vi "get_stage_position.vi"(8 "error IN":errorcluster, 11 "reference IN":refnum<k7>) -> (0 "error OUT":errorcluster, 2 "Stage position OUT":T1, 3 "reference OUT":refnum<k7>)   [LabVIEW 2020]
uses:
  typedefs/typedef_stage_position.ctl
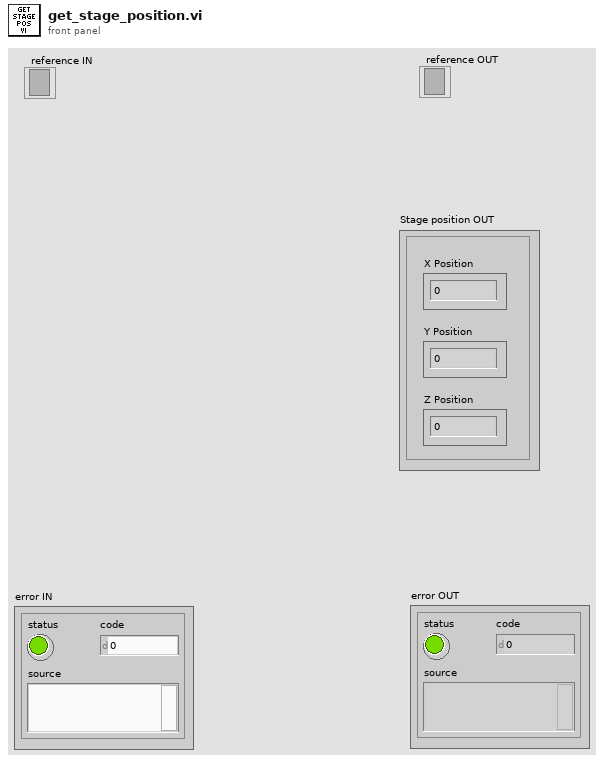
[diagram p1: front panel]
types:
  T1 = typedef "typedef_stage_position.ctl" = cluster{"X Position":dbl, "Y Position":dbl, "Z Position":dbl}
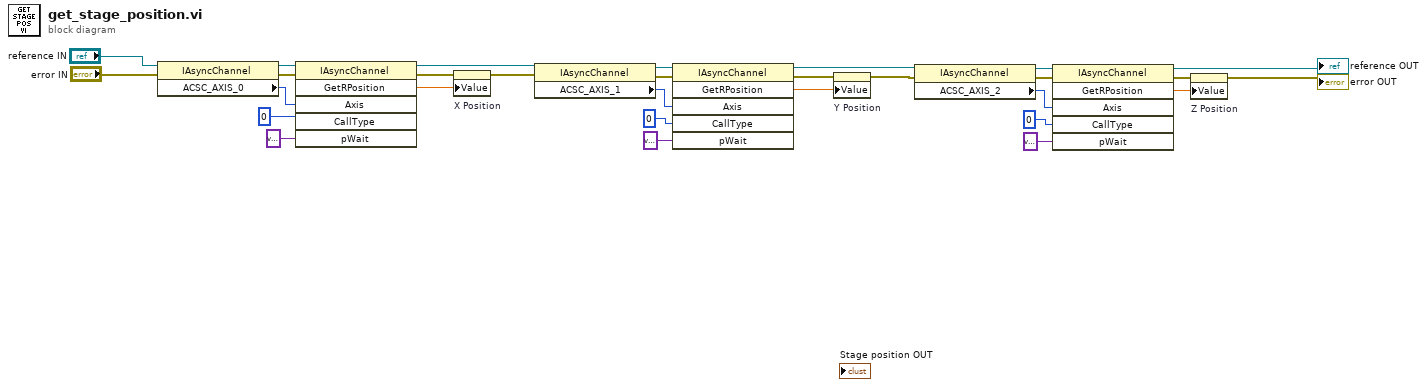
[diagram p0: block diagram]
diagram:
  n1 = property class="IAsyncChannel"(reference="reference IN", error in="error IN") -> (reference out=w29:refnum<k7>, error out=w28:errorcluster, "ACSC_AXIS_0"=w5:i32)
  n2 = invoke class="IAsyncChannel" method="GetRPosition"(reference=w29, error in=w28, "Axis"=w5, "CallType"=u64 0, "pWait"=variant) -> (reference out=w20:refnum<k7>, error out=w13:errorcluster, "GetRPosition"=w11:dbl)  [unwired: 1 in, 3 out]
  n3 = property on="X Position" class="DigNum (strict)"(error in=w13, "Value"=w11) -> (error out=w12:errorcluster)  [unwired: 1 in, 1 out]
  n4 = property class="IAsyncChannel"(reference=w20, error in=w12) -> (reference out=w25:refnum<k7>, error out=w24:errorcluster, "ACSC_AXIS_1"=w21:i32)
  n5 = invoke class="IAsyncChannel" method="GetRPosition"(reference=w25, error in=w24, "Axis"=w21, "CallType"=u64 0, "pWait"=variant) -> (reference out=w14:refnum<k7>, error out=w10:errorcluster, "GetRPosition"=w8:dbl)  [unwired: 1 in, 3 out]
  n6 = property on="Y Position" class="DigNum (strict)"(error in=w10, "Value"=w8) -> (error out=w9:errorcluster)  [unwired: 1 in, 1 out]
  n7 = property class="IAsyncChannel"(reference=w14, error in=w9) -> (reference out=w19:refnum<k7>, error out=w18:errorcluster, "ACSC_AXIS_2"=w15:i32)
  n8 = invoke class="IAsyncChannel" method="GetRPosition"(reference=w19, error in=w18, "Axis"=w15, "CallType"=u64 0, "pWait"=variant) -> (reference out=→"reference OUT":refnum<k7>, error out=w7:errorcluster, "GetRPosition"=w6:dbl)  [unwired: 1 in, 3 out]
  n9 = property on="Z Position" class="DigNum (strict)"(error in=w7, "Value"=w6) -> (error out=→"error OUT":errorcluster)  [unwired: 1 in, 1 out]
